vi "INS_civitanavi_read_PXI_subvi.vi"(11 "U8_Input":u8[](array[numeric])) -> (0 "Opp_Mode 2":string, 1 "Long_Lat_Alt":sgl[](array[numeric]), 2 "XYZ - rate":sgl[](array[numeric]), 3 "Euler Angles":sgl[](array[numeric]), 4 "GC_Counter 2":u32, 5 "CFN-IMU data":sgl[](array[numeric]), 6 "CRC?":bool)   [LabVIEW 2017]
panel:
  out "XYZ - accel":sgl[](array[numeric])
  out "INS_R":bool
  out "CRC Out":u16 format="%.0x"
  out "CRC_Input":u16 format="%x"
  out "LPI-X_R":sgl(slide)=-2.8742945e-05 scale=-6.0..6.0
  out "LPI-Y_R":sgl(slide)=-2.8742945e-05 scale=-6.0..6.0
  out "LPI-Z_R":sgl(slide)=-2.8742945e-05 scale=-6.0..6.0
  out "Longitude_R":sgl(slide)=-2.8742945e-05 scale=-180.0..180.0
  out "Altitude_R":sgl(slide)=-2.8742945e-05 scale=0.0..500.0
  out "Latitude_R":sgl(slide)=-2.8742945e-05 scale=-90.0..90.0
  out "Z_Accel_R":sgl(slide)=-2.8742945e-05 scale=-200.0..200.0
  out "X_Accel_R":sgl(slide)=-2.8742945e-05 scale=-200.0..200.0
  out "Y_Accel_R":sgl(slide)=-2.8742945e-05 scale=-200.0..200.0
  out "Z_Rate_R":sgl(slide)=-2.8742945e-05 scale=-300.0..300.0
  out "Y_ Rate_R":sgl(slide)=-2.8742945e-05 scale=-300.0..300.0
  out "X_Rate _R":sgl(slide)=-2.8742945e-05 scale=-300.0..300.0
  out "Yaw_R":sgl(slide)=-2.8742945e-05 scale=-180.0..180.0
  out "Pitch_R":sgl(slide)=-2.8742945e-05 scale=-90.0..90.0
  out "Roll_R":sgl(slide)=-2.8742945e-05 scale=-180.0..180.0
  out "Data Validity Time":u16[](array[numeric])
  out "Read String":string
  out "reserved 14":bool
  out "reserved 15":bool
  out "GC restarted 2":bool
  out "reserved 16":bool
  out "Init Align. M_Comp 2":bool
  out "Tick_Counter 2":u16
  out "Align_Word_Byte":bool[](array[boolean])
  out "GC Align Counter (s) 2":bool[](array[boolean])
  out "Fault_Code_HW 2":string
  out "ASE warning   2":bool
  out "Power warning 2":bool
  out "Motion Detection 2":bool
  out "RESERVED 4":bool
  out "RESERVED 5":bool
  out "RESERVED 6":bool
  out "Fault_Code 2":bool[](array[boolean])
  out "Operative_Mode 2":bool[](array[boolean])
  out "Op_Word_Byte":bool[](array[boolean])
  out "CRC_MSB 2":u8
  out "CRC_LSB 2":u8
  out "Status_Word_Byte":bool[](array[boolean])
  out "Data_Validity_Byte":bool[](array[boolean])
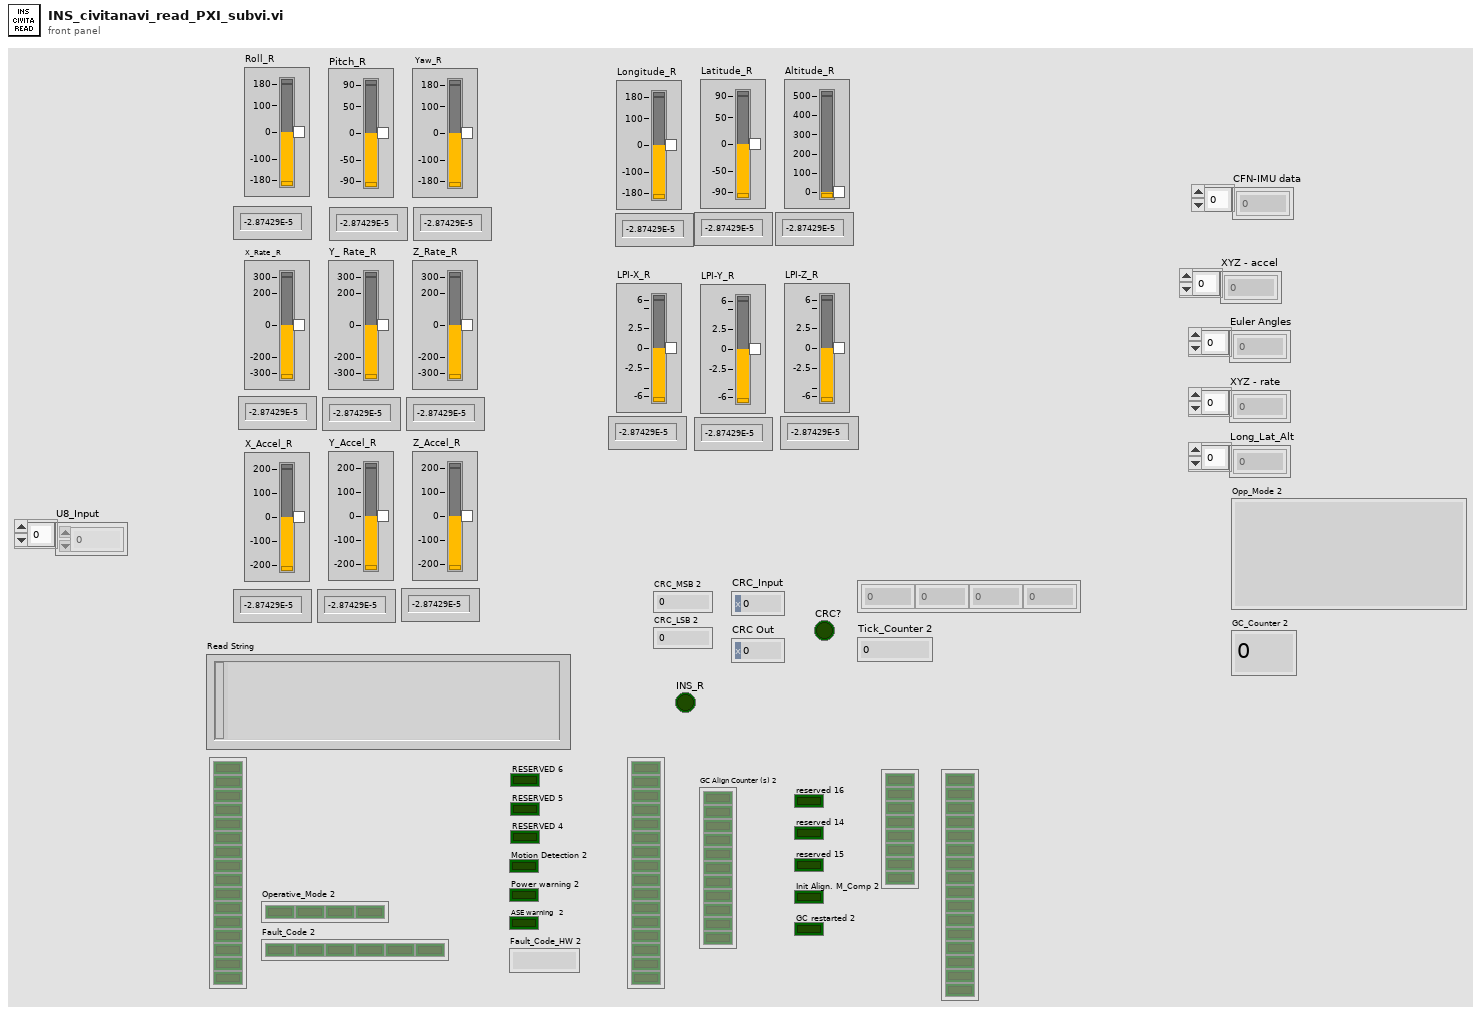
[diagram p1: front panel]
types:
  T1 = cluster{"Roll_":sgl, "Pitch_":sgl, "Yaw_":sgl, "X_Rate":sgl, "Y_ Rate":sgl, "Z_Rate":sgl, "X_Accel":sgl, "Y_Accel":sgl, "Z_Accel":sgl, "Longitude":sgl, "Latitude":sgl, "Altitude":sgl, "LPI-X":sgl, "LPI-Y":sgl, "LPI-Z":sgl}
  T2 = cluster{"Op_Word_Byte":bool[], "Opp_Mode":string, "Operative_Mode":bool[], "RESERVED":bool, "RESERVED":bool, "RESERVED":bool, "Motion Detection":bool, "Power Warning":bool, "ASE Warning":bool, "Fault_Code":bool[], "Fault_Code_HW":string}
  T3 = cluster{"Align_Word_Byte":bool[], "GC Align Counter (s)":bool[], "GC_Counter":u32, "reserved":bool, "reserved":bool, "reserved":bool, "Init Align. M_Comp":bool, "GC restarted ":bool}
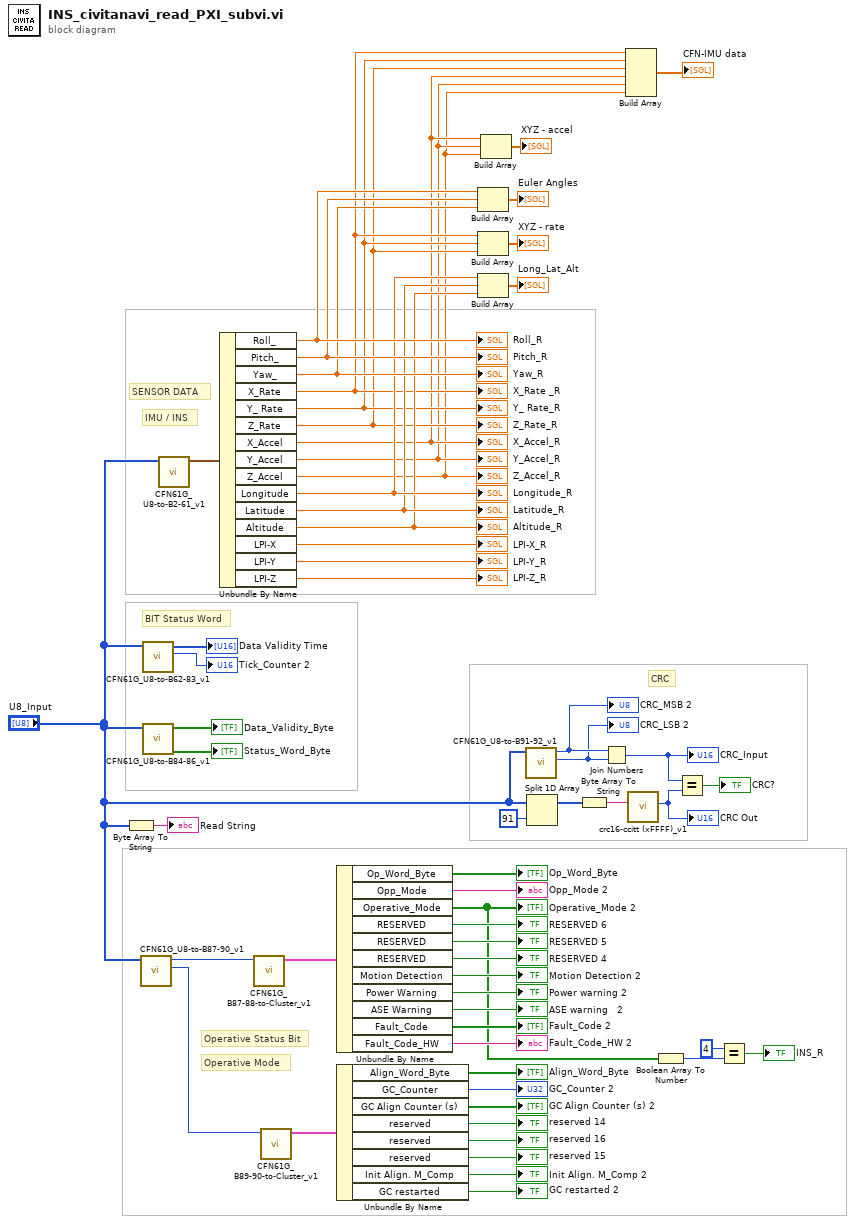
[diagram p0: block diagram]
diagram:
  # "Operative Mode"
  # "CRC"
  # "Operative Status Bit"
  # "BIT Status Word"
  # "IMU / INS"
  # "SENSOR DATA"
  n1 = Byte Array To String(unsigned byte array="U8_Input") -> (string=→"Read String":string)
  n2 = call "CFN61G_U8-to-B87-90_v1.vi"("U8_Input"="U8_Input") -> ("Align_Word"=w53:u16, "Op_Word"=w42:u16)  [unwired: 9 in]
  n3 = call "CFN61G_U8-to-B62-83_v1.vi"("U8_Input"="U8_Input") -> ("Tick_Counter"=→"Tick_Counter 2":u16, "Data Validity Time"=→"Data Validity Time":u16[])  [unwired: 8 in, 1 out]
  n4 = call "CFN61G_U8-to-B84-86_v1.vi"("U8_Input"="U8_Input") -> ("Status_Word_Byte"=→"Status_Word_Byte":bool[], "Data_Validity_Byte"=→"Data_Validity_Byte":bool[])  [unwired: 7 in, 2 out]
  n5 = call "CFN61G_U8-to-B2-61_v1.vi"("U8_Input"="U8_Input") -> ("Output_Cluster"=w31:T1)  [unwired: 10 in]
  n6 = Unbundle By Name(w31) -> ("Roll_"=w17:sgl, "Pitch_"=w16:sgl, "Yaw_"=w15:sgl, "X_Rate"=w7:sgl, "Y_ Rate"=w6:sgl, "Z_Rate"=w5:sgl, "X_Accel"=w4:sgl, "Y_Accel"=w3:sgl, "Z_Accel"=w2:sgl, "Longitude"=w13:sgl, "Latitude"=w12:sgl, "Altitude"=w11:sgl, "LPI-X"=→"LPI-X_R":sgl, "LPI-Y"=→"LPI-Y_R":sgl, "LPI-Z"=→"LPI-Z_R":sgl)
  "Roll_R" <- w17
  "Pitch_R" <- w16
  "Yaw_R" <- w15
  "X_Rate _R" <- w7
  "Y_ Rate_R" <- w6
  "Z_Rate_R" <- w5
  "Y_Accel_R" <- w3
  "X_Accel_R" <- w4
  "Z_Accel_R" <- w2
  "Latitude_R" <- w12
  "Altitude_R" <- w11
  "Longitude_R" <- w13
  n7 = call "CFN61G_B87-88-to-Cluster_v1.vi"("Op_Word"=w42) -> ("output cluster"=w41:T2)  [unwired: 10 in]
  n8 = call "CFN61G_B89-90-to-Cluster_v1.vi"("Align_Word"=w53) -> ("Cluster"=w40:T3)  [unwired: 10 in]
  n9 = Unbundle By Name(w41) -> ("Op_Word_Byte"=→"Op_Word_Byte":bool[], "Opp_Mode"=→"Opp_Mode 2":string, "Operative_Mode"=w22:bool[], "RESERVED"=→"RESERVED 6":bool, "RESERVED"=→"RESERVED 5":bool, "RESERVED"=→"RESERVED 4":bool, "Motion Detection"=→"Motion Detection 2":bool, "Power Warning"=→"Power warning 2":bool, "ASE Warning"=→"ASE warning   2":bool, "Fault_Code"=→"Fault_Code 2":bool[], "Fault_Code_HW"=→"Fault_Code_HW 2":string)
  "Operative_Mode 2" <- w22
  n10 = Unbundle By Name(w40) -> ("Align_Word_Byte"=→"Align_Word_Byte":bool[], "GC_Counter"=→"GC_Counter 2":u32, "GC Align Counter (s)"=→"GC Align Counter (s) 2":bool[], "reserved"=→"reserved 14":bool, "reserved"=→"reserved 16":bool, "reserved"=→"reserved 15":bool, "Init Align. M_Comp"=→"Init Align. M_Comp 2":bool, "GC restarted"=→"GC restarted 2":bool)
  n11 = Build Array(w17, w16, w15) -> (→"Euler Angles":sgl[])
  n12 = Build Array(w7, w6, w5) -> (→"XYZ - rate":sgl[])
  n13 = Build Array(w13, w12, w11) -> (→"Long_Lat_Alt":sgl[])
  n14 = Build Array(w4, w3, w2) -> (→"XYZ - accel":sgl[])
  n15 = call "CFN61G_U8-to-B91-92_v1.vi"("U8_Injput"="U8_Input") -> ("CRC_LSB"=w23:u8, "CRC_MSB"=w24:u8)  [unwired: 9 in]
  "CRC_LSB 2" <- w23
  "CRC_MSB 2" <- w24
  n16 = Split 1D Array(array="U8_Input", index=91) -> (first subarray=w29:u8[])  [unwired: 1 out]
  n17 = Byte Array To String(unsigned byte array=w29) -> (string=w28:string)
  n18 = Join Numbers(hi=w24, lo=w23) -> ((hi.lo)=w27:u16)
  "CRC_Input" <- w27
  n19 = Build Array(w7, w6, w5, w4, w3, w2) -> (→"CFN-IMU data":sgl[])
  n20 = call "crc16-ccitt (xFFFF)_v1.vi"("Message"=w28) -> ("CRC"=w26:u16)  [unwired: 9 in, 1 out]
  "CRC Out" <- w26
  n21 = Boolean Array To Number(Boolean array=w22) -> (number=w21:u32)
  n22 = Equal?(x=w27, y=w26) -> (x = y?=→"CRC?":bool)
  n23 = Equal?(x=u32 4, y=w21) -> (x = y?=→"INS_R":bool)
